vi "Get Enum Field Info.vi"(8 "error in (no error)":errorcluster, 11 "Enum Field ref in":u64) -> (0 "error out":errorcluster, 2 "Field Info":T1, 3 "Enum Field ref out":u64)   [LabVIEW 2019, in "gRPC Template Creation Utility.lvlib"]
uses:
  gRPC Template Creation Utility.lvlib
  TypeDefs/Enum Metadata (Scripting).ctl
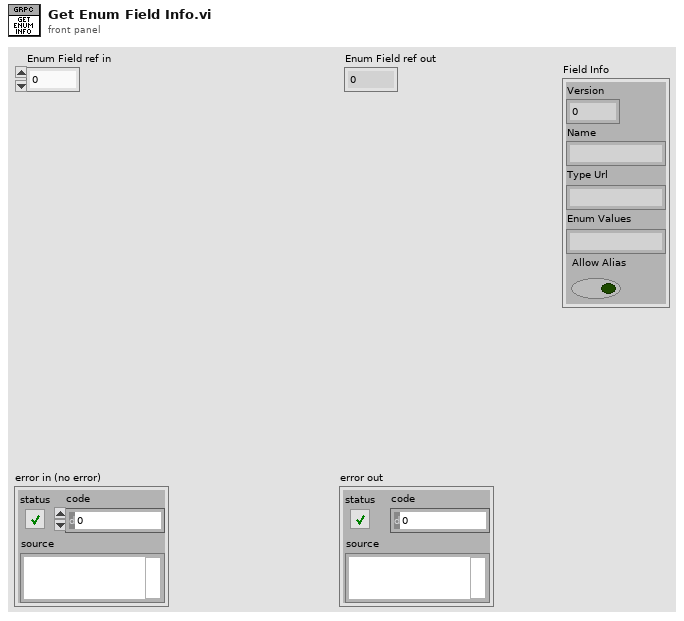
[diagram p1: front panel]
types:
  T1 = typedef "gRPC Template Creation Utility.lvlib/Enum Metadata (Scripting).ctl" = cluster{"Version":i32, "Name":string, "Type Url":string, "Enum Values":string, "Allow Alias":bool}
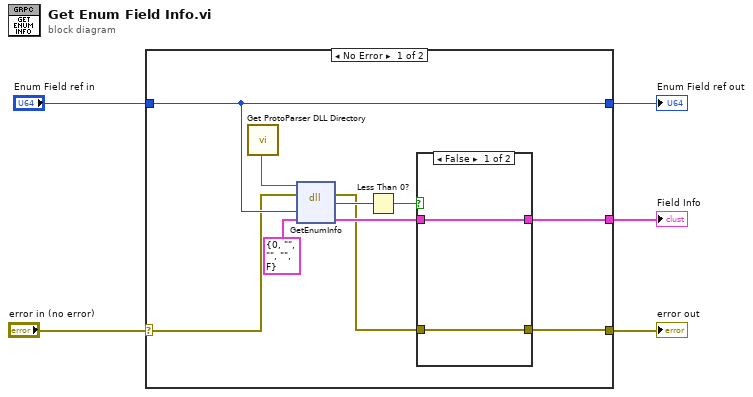
[diagram p0: block diagram]
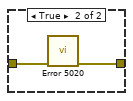
[diagram p2: hidden frame]
diagram:
  n1 = case shown="No Error" "error in (no error)" {
    selector: "error in (no error)" -> [w14 w21]
    tunnel: "Enum Field ref in" -> [w15 w20]
    tunnel: [w15 w20] -> w3
    tunnel: [w6 w21] -> w2
    tunnel: [w10 _] -> w1
    frame No Error {
      n2 = call "Get ProtoParser DLL Directory.vi"() -> ("Proto Parser Directory"=w12:path)
      n3 = dll-call lib="C:/Source/grpc-labview/labview source/Client Server Support New/gRPC Scripting Tools/Proto Parser API/Libraries/Win32/labview_grpc_generator.dll" fn="GetEnumInfo"(path in=w12, error in=w14, "field"=w15, "fieldInfo"=T1 {"Version"=0, "Name"="", "Type Url"="", "Enum Values"="", "Allow Alias"=FALSE} ("MessageElementMetadata")) -> (error out=w7:errorcluster, "return type"=w9:i32, "fieldInfo"=w11:T1)  [unwired: 2 in, 1 out]
      n4 = Less Than 0?(x=w9) -> (x < 0?=w8:bool)
      n5 = case shown="False" w8 {
        tunnel: w11 -> [w16 _]
        tunnel: [w16 _] -> w10
        tunnel: w7 -> [w17 w19]
        tunnel: [w17 w18] -> w6
        frame False {
        }
        frame True {
          n6 = call "Error 5020.vi"("error in (no error)"=w19) -> ("error out"=w18:errorcluster)  [unwired: 10 in]
        }
      }
    }
    frame Error {
    }
  }
  "Enum Field ref out" <- w3
  "error out" <- w2
  "Field Info" <- w1
